vi "create_subarray (SubVI).vi"(10 "index":i32, 11 "value":dbl) -> (3 "output array":dbl[](array[numeric]))   [LabVIEW 2014]
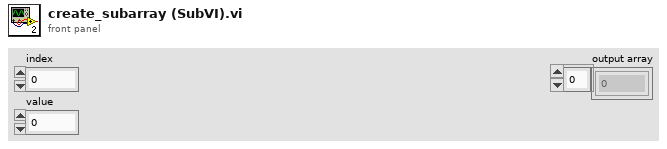
[diagram p1: front panel]
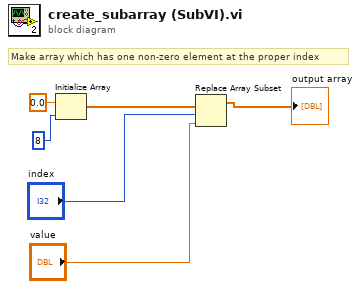
[diagram p0: block diagram]
diagram:
  # "Make array which has one non-zero element at the proper index"
  n1 = Initialize Array(0.0 ("element"), 8 ("dimension size")) -> (w4:dbl[])
  n2 = Replace Array Subset(array=w4, new element="value", index="index") -> (→"output array":dbl[])
